vi "Test PSD.vi"() -> ()   [LabVIEW 2015]
uses:
  Math VIs/LinSpace (x0-dx-npts).vi
  <vilib>/addons/Time Series Analysis/Correlation and Spectral Analysis.llb/TSA Welch (Array).vi
  Math VIs/Linear to dB (array).vi
  Conversion VIs/Create Waveform Cluster (1D).vi
  <vilib>/addons/_Advanced Signal Processing/NI_AdvSigProcTSA.lvlib
panel:
  out "Waveform Graph 2":cluster{dbl, "dx":dbl, "Y":dbl[]}[](graph)
  out "Waveform Graph":dbl[][](graph)
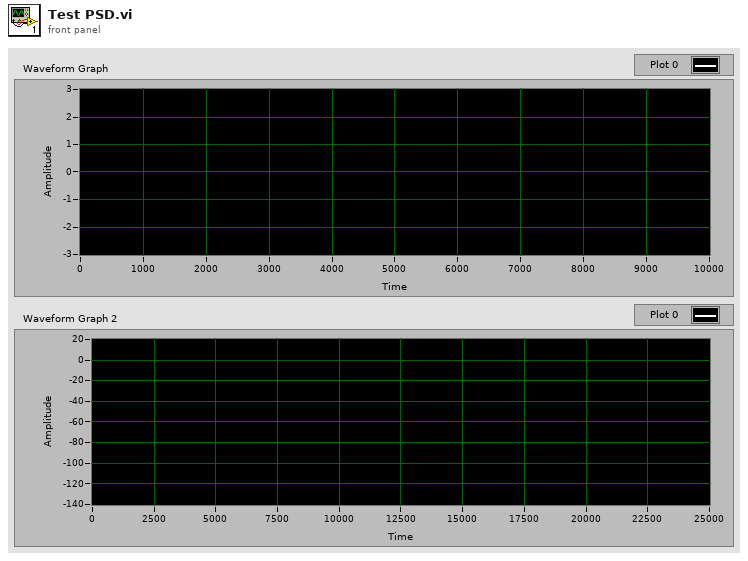
[diagram p1: front panel]
types:
  T1 = cluster{"window":u16, "length":i32, "overlap (%)":dbl}
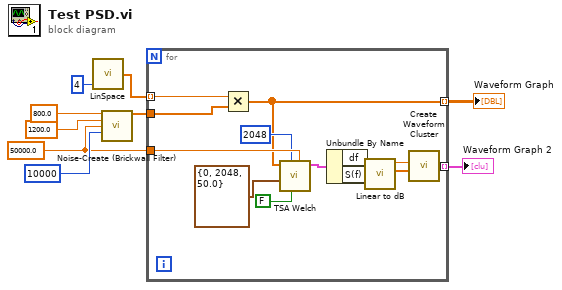
[diagram p0: block diagram]
diagram:
  w5 = 50000.0 ("Sampling rate (Hz)")
  n1 = call-poly "LinSpace.vi"("npts"=4) -> ("Array"=w1:dbl[])  [unwired: 3 in, 1 out]
  n2 = call "Noise-Create (Brickwall Filter).vi"("Min Frequency (Hz)"=800.0, "Max Frequency (Hz)"=1200.0, "Sampling rate (Hz)"=w5, "Length (points)"=10000) -> ("Filtered Noise"=w6:dbl[])  [unwired: 9 in, 2 out]
  n3 = for {
    tunnel: w6 -> [w21]
    tunnel: w5 -> [w20]
    tunnel: [w14] -> w4 mode=indexing
    tunnel: [w12] -> w3 mode=indexing
    tunnel: w1 -> [w11] mode=indexing
    n4 = Multiply(x=w11, y=w21) -> (x*y=w12:dbl[])
    n5 = call-poly <vilib>:"TSA Welch.vi"("sampling rate"=w20, "dB on? (T)"=FALSE, "frequency bins"=2048, "window info"=T1 {"window"=0, "length"=2048, "overlap (%)"=50.0}, "Xt"=w12) -> ("PSD"=w17:cluster{"f0":dbl, "df":dbl, "S(f)":dbl[]})  [unwired: 5 in, 1 out]
    n6 = Unbundle By Name(w17) -> ("df"=w16:dbl, "S(f)"=w15:dbl[])
    n7 = call-poly "Linear to dB.vi"("linear"=w15) -> ("dB"=w10:dbl[])
    n8 = call-poly "Create Waveform Cluster.vi"("dx"=w16, "Y"=w10) -> ("waveform cluster"=w14:cluster{dbl, "dx":dbl, "Y":dbl[]})  [unwired: 3 in]
  }
  "Waveform Graph" <- w3
  "Waveform Graph 2" <- w4
